vi "get data definition.vi"(10 "channel classification":T1, 11 "System Diagnostics runtime in":refnum<class "System Diagnostics runtime.lvclass">) -> (1 "valid?":bool, 2 "index cluster":variant, 3 "System Diagnostics runtime out":refnum<class "System Diagnostics runtime.lvclass">)   [LabVIEW 2013, in "System Diagnostics runtime.lvclass"]
uses:
  System Diagnostics runtime.lvclass
  <vilib>/NI/Tag Bus Module Framework/channel/channel classification.ctl
  input user data.ctl
  <vilib>/NI/Tag Bus Module Framework/channel/TBM channel.lvclass
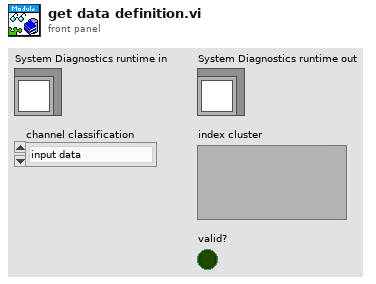
[diagram p1: front panel]
types:
  T1 = typedef "TBM channel.lvclass/channel classification.ctl" = enum16{"input data", "output data", "processing parameter", "processing result"}
  T2 = typedef "System Diagnostics runtime.lvclass/input user data.ctl" = cluster{"CPU load average":dbl, "timed structures load":dbl, "free memory":dbl, "contiguous memory":dbl}
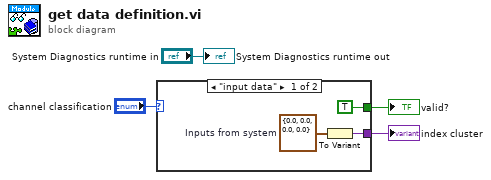
[diagram p0: block diagram]
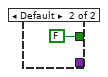
[diagram p2: hidden frame]
diagram:
  n1 = case shown="\"input data\"" "channel classification" {
    tunnel: [TRUE FALSE] -> w2
    tunnel: [w6 _] -> w1
    frame "input data" {
      w7 = T2 {"CPU load average"=0.0, "timed structures load"=0.0, "free memory"=0.0, "contiguous memory"=0.0}  # Inputs from system
      n2 = To Variant(anything=w7) -> (Variant=w6:variant)
    }
    frame Default {
    }
  }
  "valid?" <- w2
  "index cluster" <- w1
  "System Diagnostics runtime out" <- "System Diagnostics runtime in"
